vi "Perfs.vi"() -> ()   [LabVIEW 2024]
uses:
  POTBuffer/Tests/Perf/POTTypedCircularBuffer.Tests.Perf.lvlib
  TypedCircularBuffer/Tests/Perf/TypedCircularBuffer.Tests.Perf.lvlib
  VarCircularBuffer/Tests/Perf/VarCircularBuffer.Tests.Perf.lvlib
  RotateCircularBuffer/Tests/Perf/RotateCircularBuffer.Tests.Perf.lvlib
  RefTypedCircularBuffer/Tests/Perf/RefTypedCircularBuffer.Tests.Perf.lvlib
  MalleableCircularBuffer/Tests/Perf/CircularBuffer.Test.Perf.lvlib
panel:
  out "Malleable":dbl format="%#_6p"
  out "Queue":dbl format="%#_6p"
  out "Rotate":dbl format="%#_6p"
  out "Variant":dbl format="%#_6p"
  out "Typed Any Size":dbl format="%#_6p"
  out "Typed POT":dbl format="%#_6p"
  # "Note this is for simple (int) data type complex data type will like render different results"
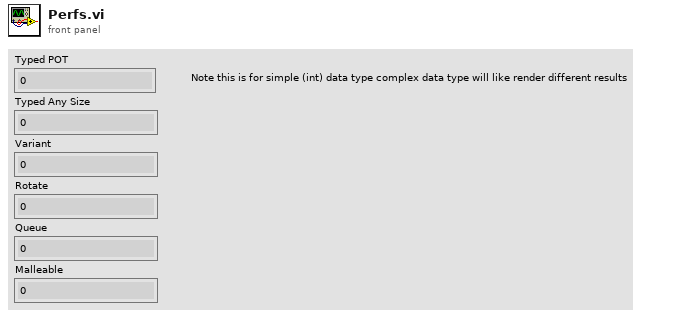
[diagram p1: front panel]
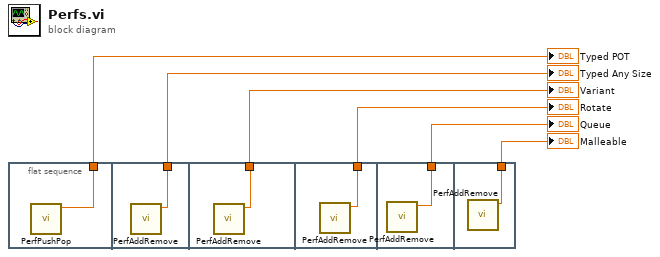
[diagram p0: block diagram]
diagram:
  n1 = flat-sequence {
    tunnel: [w7] -> w6
    tunnel: [w8] -> w5
    tunnel: [w9] -> w4
    tunnel: [w10] -> w3
    tunnel: [w11] -> w2
    tunnel: [w12] -> w1
    frame #0 {
      n2 = call "PerfPushPop.vi"() -> ("Add mean"=w7:dbl)  [unwired: 11 in]
    }
    frame #1 {
      n3 = call "PerfAddRemove.vi"() -> ("Add mean"=w8:dbl)  [unwired: 11 in]
    }
    frame #2 {
      n4 = call "PerfAddRemove.vi"() -> ("Add time"=w9:dbl)  [unwired: 11 in]
    }
    frame #3 {
      n5 = call "PerfAddRemove.vi"() -> ("Add time"=w10:dbl)  [unwired: 11 in]
    }
    frame #4 {
      n6 = call "PerfAddRemove.vi"() -> ("Add time"=w11:dbl)  [unwired: 11 in]
    }
    frame #5 {
      n7 = call "PerfAddRemove.vi"() -> ("Add time"=w12:dbl)  [unwired: 11 in]
    }
  }
  "Typed POT" <- w6
  "Typed Any Size" <- w5
  "Variant" <- w4
  "Rotate" <- w3
  "Queue" <- w2
  "Malleable" <- w1
